vi "GenTimeVector.vi"(8 "error in (no error)":errorcluster, 9 "Offset":dbl, 10 "Multiplier - dT":dbl, 11 "# of elements":dbl) -> (0 "error out":errorcluster, 3 "Time Vector":dbl[][](array[numeric]))   [LabVIEW 2018, in "DisplayWaveform.lvlib" / "DisplayWaveforms.lvclass"]
doc: "Generate Time Vector. Returns a 2D array with first column as the Time vector."
uses:
  DisplayWaveforms.lvclass
  <vilib>/Analysis/NI_AALBase.lvlib
  <vilib>/Analysis/1siggen.llb/Ramp Pattern by Delta.vi
panel:
  # "For instructions on how to use the JKI State Machine Objects, examples and video tutorials, visit:\nhttp://jki.net/state-machine-objects/\n\nJKI State Machine Objects™\nhttp://jki.net/state-machine-objects/\nCopyright (C) 2005-2015, JKI <info@jki.net>\nALL RIGHTS RESERVED"
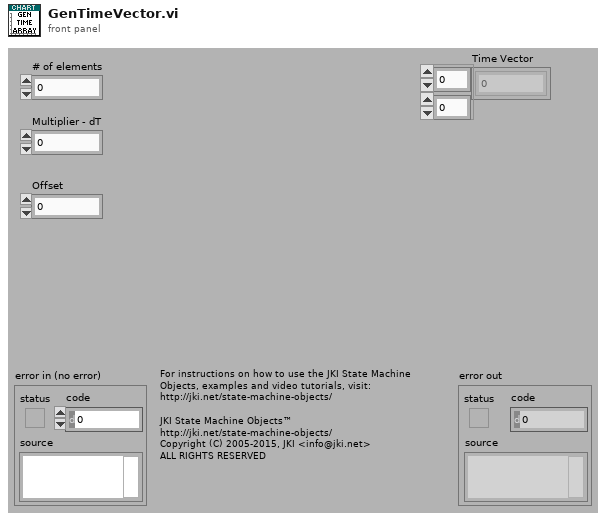
[diagram p1: front panel]
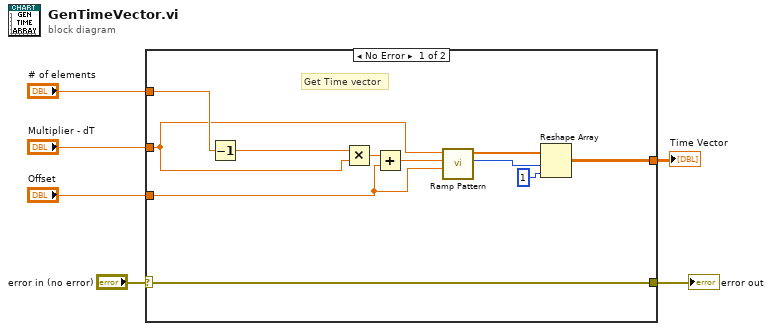
[diagram p0: block diagram]
diagram:
  n1 = case shown="No Error" "error in (no error)" {
    selector: "error in (no error)" -> [w17 w18]
    tunnel: [w17 w18] -> w6
    tunnel: "# of elements" -> [w10 _]
    tunnel: "Multiplier - dT" -> [w9 _]
    tunnel: "Offset" -> [w8 _]
    tunnel: [w7 _] -> w1
    frame No Error {
      # "Get Time vector"
      n2 = Decrement(x=w10) -> (x-1=w15:dbl)
      n3 = Multiply(x=w15, y=w9) -> (x*y=w14:dbl)
      n4 = Add(x=w14, y=w8) -> (x+y=w13:dbl)
      n5 = call-poly <vilib>:"Ramp Pattern.vi"("start"=w8, "end"=w13, "delta"=w9) -> ("samples"=w12:i32, "Ramp Pattern"=w11:dbl[])  [unwired: 6 in, 1 out]
      n6 = Reshape Array(w11, w12, 1 ("dimension size")) -> (w7:dbl[][])
    }
    frame Error {
    }
  }
  "error out" <- w6
  "Time Vector" <- w1
